vi "4461.Start.AO.vi"(8 "error in (no error)":errorcluster, 11 "Instrument.Lockin in":refnum<class "Instrument.Lockin.lvclass">) -> (0 "error out":errorcluster, 3 "Instrument.Lockin out":refnum<class "Instrument.Lockin.lvclass">)   [LabVIEW 2016, in "Instrument.Lockin.lvclass"]
uses:
  Instrument.Lockin.lvclass
  Instrument.Lockin.lvclass/Instrument.Lockin.ctl
  <vilib>/DAQmx/write.llb/DAQmx Write (Analog 1D Wfm NChan NSamp).vi
  <vilib>/DAQmx/miscellaneous.llb/DAQmx Fill In Error Info.vi
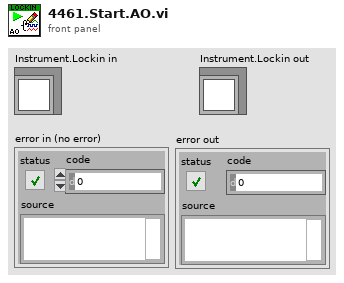
[diagram p1: front panel]
types:
  T1 = typedef "Instrument.Lockin.lvclass/AO-cluster.ctl" = cluster{"AO Amp (V)":T2, "AO DC (V)":T3, "AO f (Hz)":T4, "AO Phase (°)":T5, "Function":T6, "I+":bool[], "Sweeping":bool[]}
  T2 = typedef "Instrument.Lockin.lvclass/AO_Amp-array.ctl" = dbl[]
  T3 = typedef "Instrument.Lockin.lvclass/AO_DC-array.ctl" = dbl[]
  T4 = typedef "Instrument.Lockin.lvclass/AO_f-array.ctl" = dbl[]
  T5 = typedef "Instrument.Lockin.lvclass/AO_phi-array.ctl" = dbl[]
  T6 = typedef "Instrument.Lockin.lvclass/Function-array.ctl" = T7[]
  T7 = typedef "Instrument.Lockin.lvclass/Function-enum.ctl" = enum16{"Sine", "Triangle", "Square", "Sawtooth"}
  T8 = typedef "Instrument.Lockin.lvclass/REF-cluster.ctl" = cluster{"REF f (Hz)":T9, "REF phi (°)":T10}
  T9 = typedef "Instrument.Lockin.lvclass/REF_f-array.ctl" = dbl[]
  T10 = typedef "Instrument.Lockin.lvclass/REF_phi-array.ctl" = dbl[]
  T11 = typedef "Instrument.Lockin.lvclass/Sampling.ctl" = cluster{"Fs":dbl, "#s":i32}
  T12 = typedef "Instrument.Lockin.lvclass/DAQType-enum.ctl" = enum16{"None", "USB 4431", "PXI 446x"}
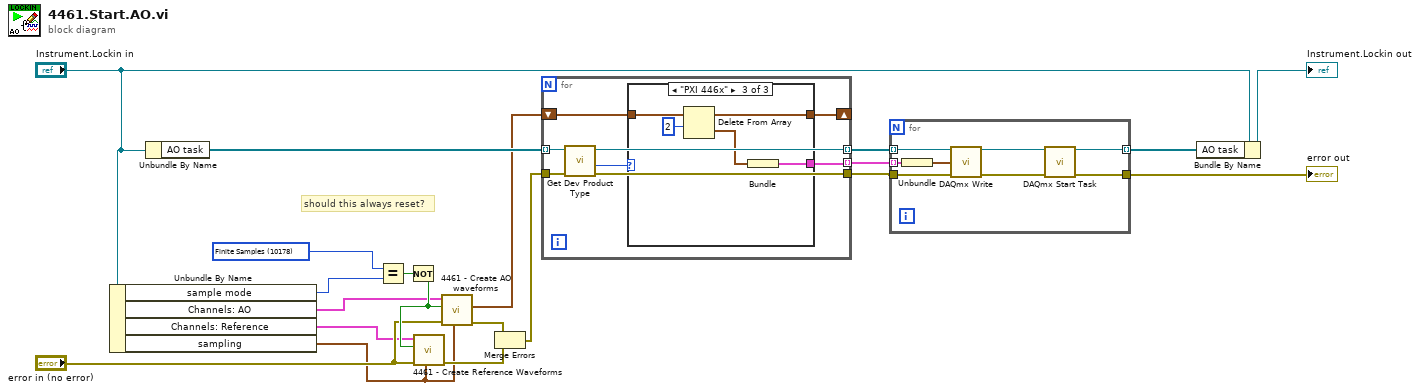
[diagram p0: block diagram]
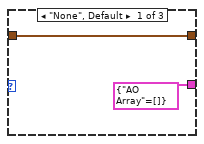
[diagram p2: hidden frame]
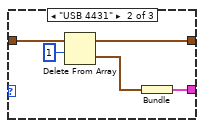
[diagram p3: hidden frame]
diagram:
  w13 = 10178 items=["Finite Samples"=10178, "Continuous Samples"=10123] ("sample mode 2")
  # "should this always reset?"
  n1 = Unbundle By Name("Instrument.Lockin in") -> ("sample mode"=w14:i32, "Channels: AO"=w16:T1, "Channels: Reference"=w15:T8, "sampling"=w3:T11)
  n2 = Unbundle By Name("Instrument.Lockin in") -> ("AO task"=w8:refnum<k21>[])
  n3 = Equal?(x=w13, y=w14) -> (x = y?=w17:bool)
  n4 = Not(x=w17) -> (.not. x?=w20:bool)
  n5 = call "4461 - Create Reference Waveforms.vi"("sampling"=w3, "error in (no error)"="error in (no error)", "reset signal"=w20, "Lockin"=w15) -> ("error out"=w19:errorcluster)  [unwired: 4 in, 3 out]
  n6 = call "4461 - Create AO waveforms.vi"("sampling"=w3, "error in (no error)"="error in (no error)", "reset signal"=w20, "AO"=w16) -> ("error out"=w2:errorcluster, "AO Array"=w7:waveform(dbl)[])  [unwired: 4 in, 2 out]
  n7 = Merge Errors(w2, w19) -> (w1:errorcluster)
  n8 = for {
    tunnel: w8 -> [w28] mode=indexing
    shift-right: [w25] -> _
    shift-left: w7 -> [w26]
    tunnel: [w24] -> w6 mode=indexing
    tunnel: [w23] -> w5 mode=indexing
    tunnel: w1 -> [w22]
    tunnel: [w21] -> w4
    n9 = call "Get Dev Product Type.vi"("error in (no error)"=w22, "Refnum in"=w28) -> ("error out"=w21:errorcluster, "DAQ Type"=w27:T12, "Refnum out"=w23:refnum<k21>)  [unwired: 6 in, 1 out]
    n10 = case shown="\"PXI 446x\"" w27 {
      tunnel: w26 -> [w30 w35 w40]
      tunnel: [w30 w34 w39] -> w25
      tunnel: [cluster{"AO Array":waveform(dbl)[]} {"AO Array"=[]} w32 w36] -> w24
      frame "None", Default {
      }
      frame "USB 4431" {
        n11 = Delete From Array(array=w35, length=1) -> (deleted portion=w31:waveform(dbl)[], array with subset deleted=w34:waveform(dbl)[])  [unwired: 1 in]
        n12 = Bundle("AO Array"=w31) -> (w32:cluster{"AO Array":waveform(dbl)[]})  [unwired: 1 in]
      }
      frame "PXI 446x" {
        n13 = Delete From Array(array=w40, length=2) -> (deleted portion=w37:waveform(dbl)[], array with subset deleted=w39:waveform(dbl)[])  [unwired: 1 in]
        n14 = Bundle("AO Array"=w37) -> (w36:cluster{"AO Array":waveform(dbl)[]})  [unwired: 1 in]
      }
    }
  }
  n15 = for {
    tunnel: w5 -> [w46] mode=indexing
    tunnel: w4 -> [w45]
    tunnel: [w44] -> w9
    tunnel: [w43] -> w10 mode=indexing
    tunnel: w6 -> [w42] mode=indexing
    n16 = Unbundle(w42) -> ("AO Array"=w41:waveform(dbl)[])
    n17 = call-poly <vilib>:"DAQmx Write.vi"("task/channels in"=w46, "data"=w41, "error in"=w45) -> ("task out"=w47:refnum<k21>, "error out"=w48:errorcluster)  [unwired: 10 in, 1 out]
    n18 = call <vilib>:"DAQmx Start Task.vi"("task/channels in"=w47, "error in"=w48) -> ("task out"=w43:refnum<k21>, "error out"=w44:errorcluster)  [unwired: 12 in]
  }
  "error out" <- w9
  n19 = Bundle By Name(cluster="Instrument.Lockin in", "AO task"=w10) -> (→"Instrument.Lockin out":refnum<class "Instrument.Lockin.lvclass">)
